vi "getNumberOfApplicationInstances.vi"(8 "error in (no error)":errorcluster, 11 "VGS_RemoteControlClient in":refnum<class "VGS_RemoteControlClient.lvclass">) -> (0 "error out":errorcluster, 2 "getNumberOfApplicationInstances":u32, 3 "VGS_RemoteControlClient out":refnum<class "VGS_RemoteControlClient.lvclass">)   [LabVIEW 2022 SP3, in "LV_VGS.lvlib" / "VGS_RemoteControlClient.lvclass"]
doc: "<B>Retrieves the number of applications active on the system running the RCS. </B>\n\nReturns the number of applications.\n\nEmit error RemoteControlServiceIsNotAvailableException if the remote control service doesn't run. \nEmit error UnableToGetNumberOfApplicationInstancesException if the remote control service could not determine the number of applications."
uses:
  VGS_RemoteControlClient.lvclass
  VGS_RemoteControlClient.lvclass/VGS_RemoteControlClient.ctl
  C:/Users/Andrey/Documents/GitHub/LV_VGS/vgs_project.dll
  vgs_project.dll
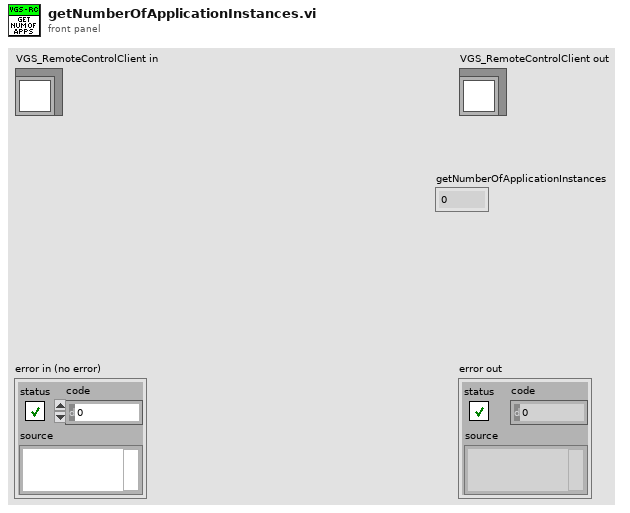
[diagram p1: front panel]
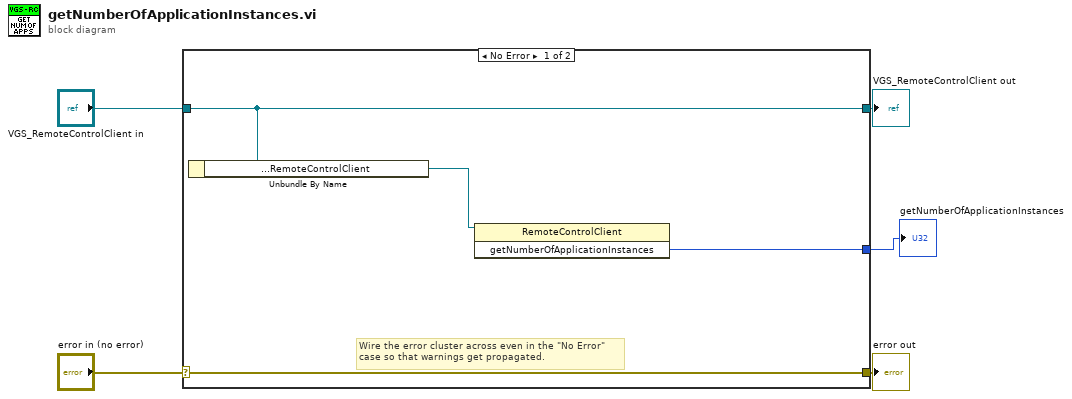
[diagram p0: block diagram]
diagram:
  n1 = case shown="No Error" "error in (no error)" {
    selector: "error in (no error)" -> [w9 w11]
    tunnel: [w9 w11] -> w4
    tunnel: [w8 w10] -> w2
    tunnel: "VGS_RemoteControlClient in" -> [w8 w10]
    tunnel: [w6 _] -> w1
    frame No Error {
      # "Wire the error cluster across even in the \"No Error\"\ncase so that warnings get propagated."
      n2 = Unbundle By Name(w8) -> ("VGS.Project.Interop.RemoteControlClient"=w7:refnum<k24>)
      n3 = invoke class="RemoteControlClient" method="getNumberOfApplicationInstances"(reference=w7) -> ("getNumberOfApplicationInstances"=w6:u32)  [unwired: 2 in, 2 out]
    }
    frame Error {
    }
  }
  "error out" <- w4
  "VGS_RemoteControlClient out" <- w2
  "getNumberOfApplicationInstances" <- w1
